vi "独立看门狗实验.vi"   [LabVIEW 2011]
uses:
  <vilib>/STM32_DriverVI_Interface_F4/WDG/IWDG_PSC_F4.ctl
  <vilib>/eio/EIO_TerminalDirection.ctl
  <vilib>/STM32_DriverVI_Interface_F4/GPIO_EIO/GPO_EIO_Inner_F4.vi
  <vilib>/STM32_DriverVI_Interface_F4/GPIO_EIO/GPI_EIO_Inner_F4.vi
  <vilib>/eio/EIONode/EIONode.xnode
types:
  T1 = typedef "IWDG_PSC_F4.ctl" = u8
  T2 = enum8{"P0", "P1", "P2", "P3", "P4", "P5", "P6", "P7", "P8", "P9", "P10", "P11", "P12", "P13", "P14", "P15"}
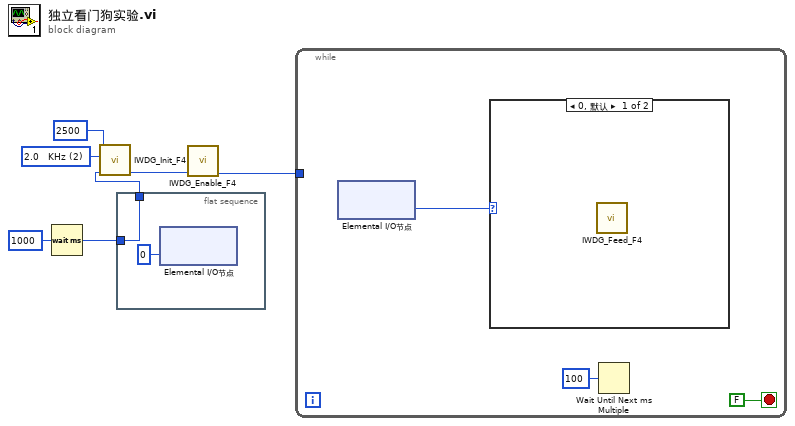
[diagram p0: block diagram]
diagram:
  w7 = T1 2 items=["8.0   KHz", "4.0   KHz", "2.0   KHz", "1.0   KHz", "500  Hz", "250  Hz", "125  Hz"] ("IWDG 预分频时基")
  n1 = Wait (ms)(milliseconds to wait=u32 1000 ("等待时间（毫秒）")) -> (millisecond timer value=w2:u32)
  n2 = call <vilib>:"IWDG_Init_F4.vi"("err_in"=w1, "IWDG 预分频时基"=w7, "自动重装值（1~4095）"=u16 2500) -> ("err_out"=w5:u8)  [unwired: 8 in]
  n3 = flat-sequence {
    tunnel: w2 -> [w8]
    tunnel: [w8] -> w1
    frame #0 {
      n4 = xnode "Elemental I/O节点"("LED_4"=u8 0) -> ()  [unwired: 1 in, 1 out]
    }
  }
  n5 = call <vilib>:"IWDG_Enable_F4.vi"("err_in"=w5) -> ("err_out"=w4:u8)  [unwired: 10 in]
  n6 = while {
    tunnel: w4 -> [_]
    stop <- FALSE stop-if-true
    n7 = xnode "Elemental I/O节点"() -> ("KEY_4"=w14:u8)  [unwired: 1 in, 1 out]
    n8 = case shown="0, 默认" w14 {
      frame 0, Default {
        n9 = call <vilib>:"IWDG_Feed_F4.vi"() -> ()  [unwired: 11 in, 1 out]
      }
      frame 1 {
      }
    }
    n10 = Wait Until Next ms Multiple(millisecond multiple=u32 100 ("毫秒倍数")) -> ()  [unwired: 1 out]
  }
